vi "CheckPassword.vi"(11 "Administrator password":string) -> (3 "Boolean":bool)   [LabVIEW 2013]
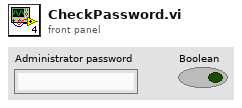
[diagram p1: front panel]
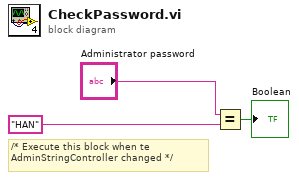
[diagram p0: block diagram]
diagram:
  # "/* Execute this block when te AdminStringController changed */"
  n1 = Equal?(x="Administrator password", y="HAN") -> (x = y?=→"Boolean":bool)
